vi "Initialize Z Stack.vi"(6 "error in (no error)":errorcluster, 8 "Zstack Settings in":T1, 9 "Automation State in":T3={"Automation State"=enum."Idle", "Handle out"=0, "ZO State"={"ZO Settings"={"Acquisition Settings"={"Save?"=FALSE, "DCIMG Path"=path "", "Filename"="", "Total Frames"=0, "Sender"=enum."UI"}, "Shift Amplitude"=0.0, "Initial Zernike Vector"=[]}, "Zernike Size"=15, "Points per order"=15, "Zernike State"=enum."Idle", "Zernike Vectors"=[], "Total Frames"=15, "Current Frame"=15}, "Zstack State"={"Zstack Settings"={"Acquisition Settings"={"Save?"=FALSE, "DCIMG Path"=path "", "Filename"="", "Total Frames"=0, "Sender"=enum."UI"}, "XYZ start"=[], "XYZ end"=[]}, "Zstack State"=enum."Idle", "Stack Coordinates"=[], "Total Frames"=15, "Current Frame"=15}}) -> (0 "error out":errorcluster, 3 "Automation State Out":T3={"Automation State"=enum."Idle", "Handle out"=0, "ZO State"={"ZO Settings"={"Acquisition Settings"={"Save?"=FALSE, "DCIMG Path"=path "", "Filename"="", "Total Frames"=0, "Sender"=enum."UI"}, "Shift Amplitude"=0.0, "Initial Zernike Vector"=[]}, "Zernike Size"=15, "Points per order"=15, "Zernike State"=enum."Idle", "Zernike Vectors"=[], "Total Frames"=15, "Current Frame"=15}, "Zstack State"={"Zstack Settings"={"Acquisition Settings"={"Save?"=FALSE, "DCIMG Path"=path "", "Filename"="", "Total Frames"=0, "Sender"=enum."UI"}, "XYZ start"=[], "XYZ end"=[]}, "Zstack State"=enum."Idle", "Stack Coordinates"=[], "Total Frames"=15, "Current Frame"=15}})   [LabVIEW 2015, in "Automation.lvlib"]
uses:
  Automation.lvlib
  Automation State.ctl
  Automation Loop State.ctl
  ZO State.ctl
  ZO Settings.ctl
  Camera/Acquisition Settings.ctl
  Zstack State.ctl
  Zstack Settings.ctl
  Camera/Camera.lvlib
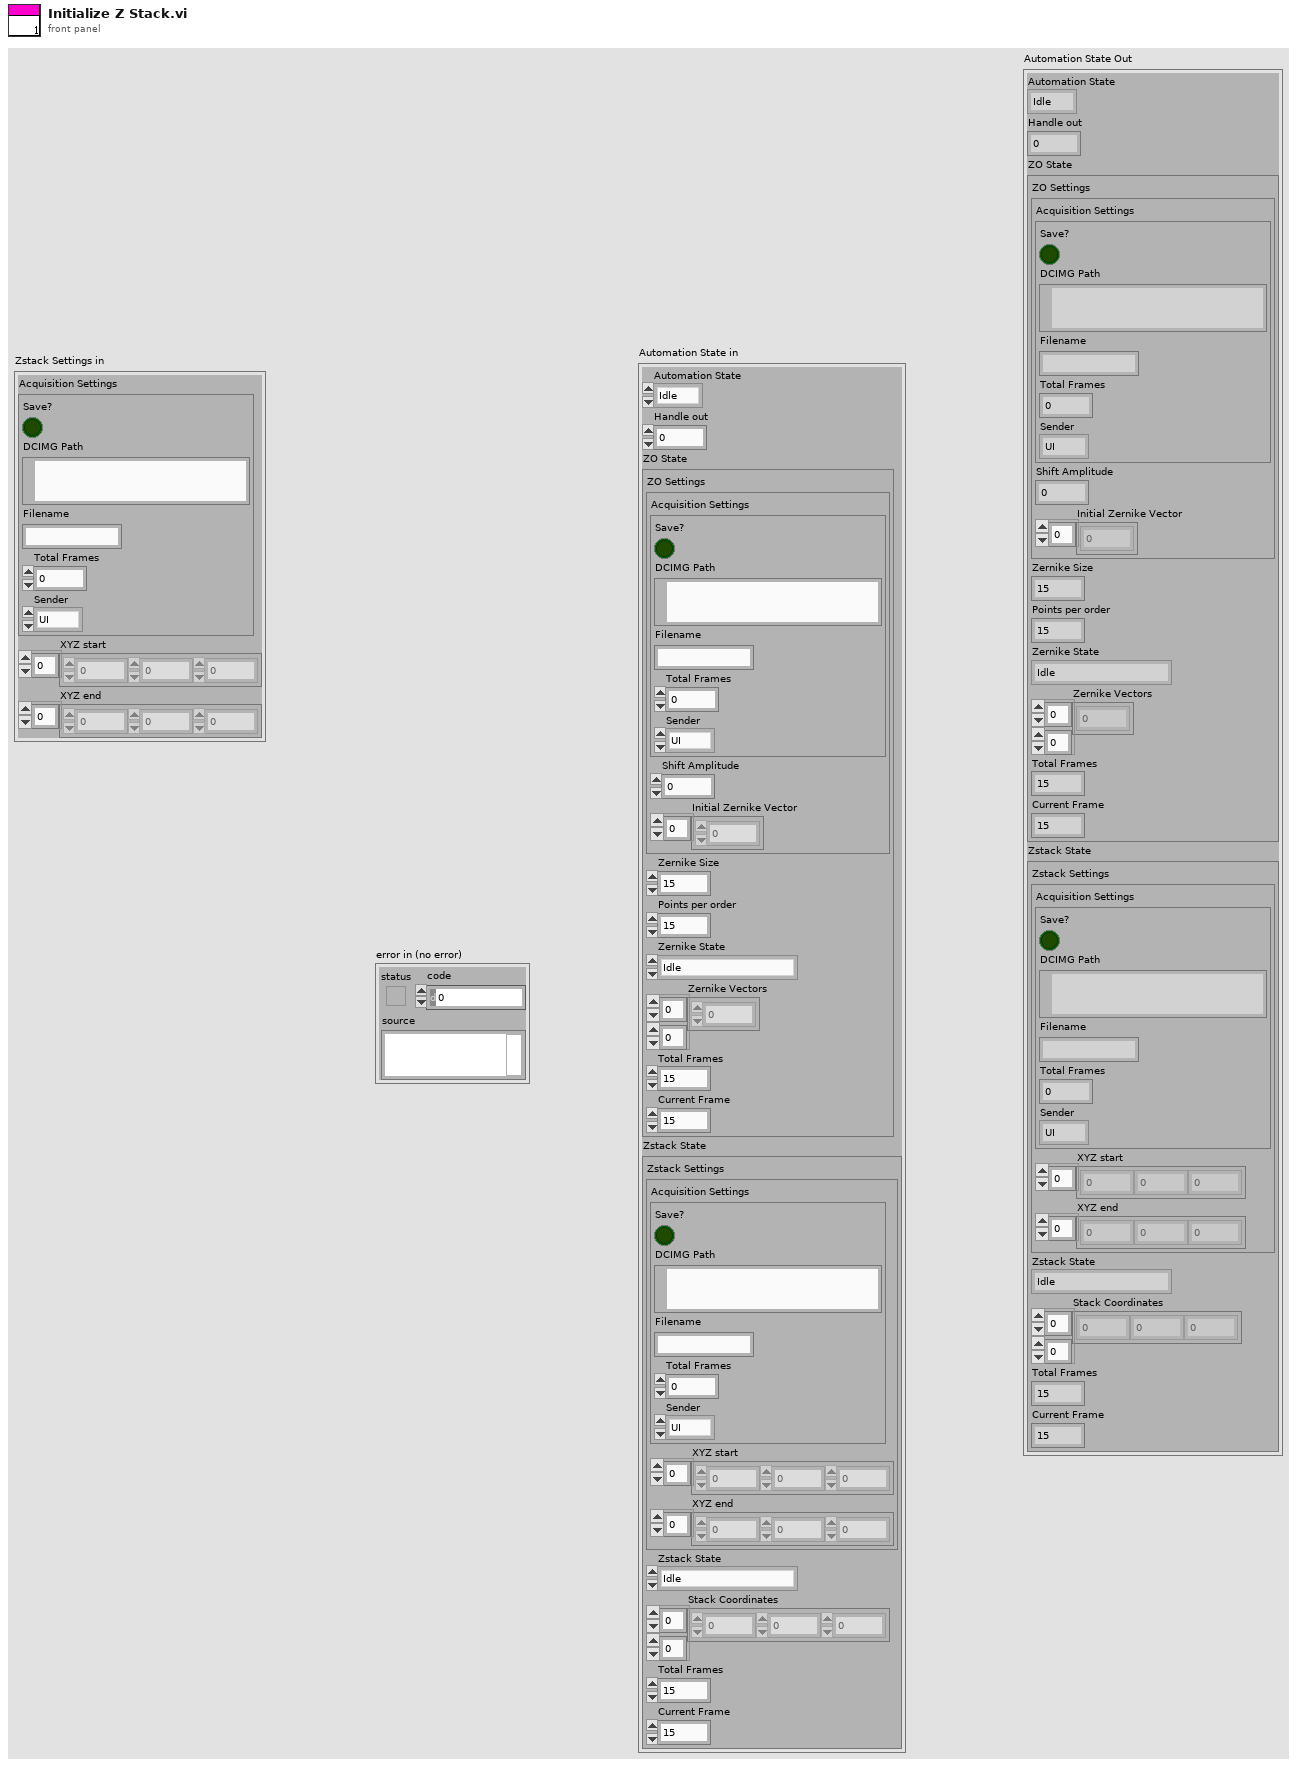
[diagram p1: front panel]
types:
  T1 = typedef "Automation.lvlib/Zstack Settings.ctl" = cluster{"Acquisition Settings":T2, "XYZ start":dbl[], "XYZ end":dbl[]}
  T2 = typedef "Camera.lvlib/Acquisition Settings.ctl" = cluster{"Save?":bool, "DCIMG Path":path, "Filename":string, "Total Frames":i32, "Sender":enum16{"UI", "Automation"}}
  T3 = typedef "Automation.lvlib/Automation State.ctl" = cluster{"Automation State":T4, "Handle out":u32, "ZO State":T5, "Zstack State":T7}
  T4 = typedef "Automation.lvlib/Automation Loop State.ctl" = enum16{"Idle", "Zernike Optimization", "Z Stack"}
  T5 = typedef "Automation.lvlib/ZO State.ctl" = cluster{"ZO Settings":T6, "Zernike Size":i32, "Points per order":i32, "Zernike State":enum16{"Idle", "Waiting for Camera Init.", "Wait for camera frame", "Ready for new mirror config"}, "Zernike Vectors":dbl[][], "Total Frames":i32, "Current Frame":i32}
  T6 = typedef "Automation.lvlib/ZO Settings.ctl" = cluster{"Acquisition Settings":T2, "Shift Amplitude":dbl, "Initial Zernike Vector":dbl[]}
  T7 = typedef "Automation.lvlib/Zstack State.ctl" = cluster{"Zstack Settings":T1, "Zstack State":enum16{"Idle", "Waiting for Camera Init.", "Wait for camera frame", "Ready for new position"}, "Stack Coordinates":dbl[][], "Total Frames":i32, "Current Frame":i32}
  T8 = enum16{"Idle", "Waiting for Camera Init.", "Wait for camera frame", "Ready for new position"}
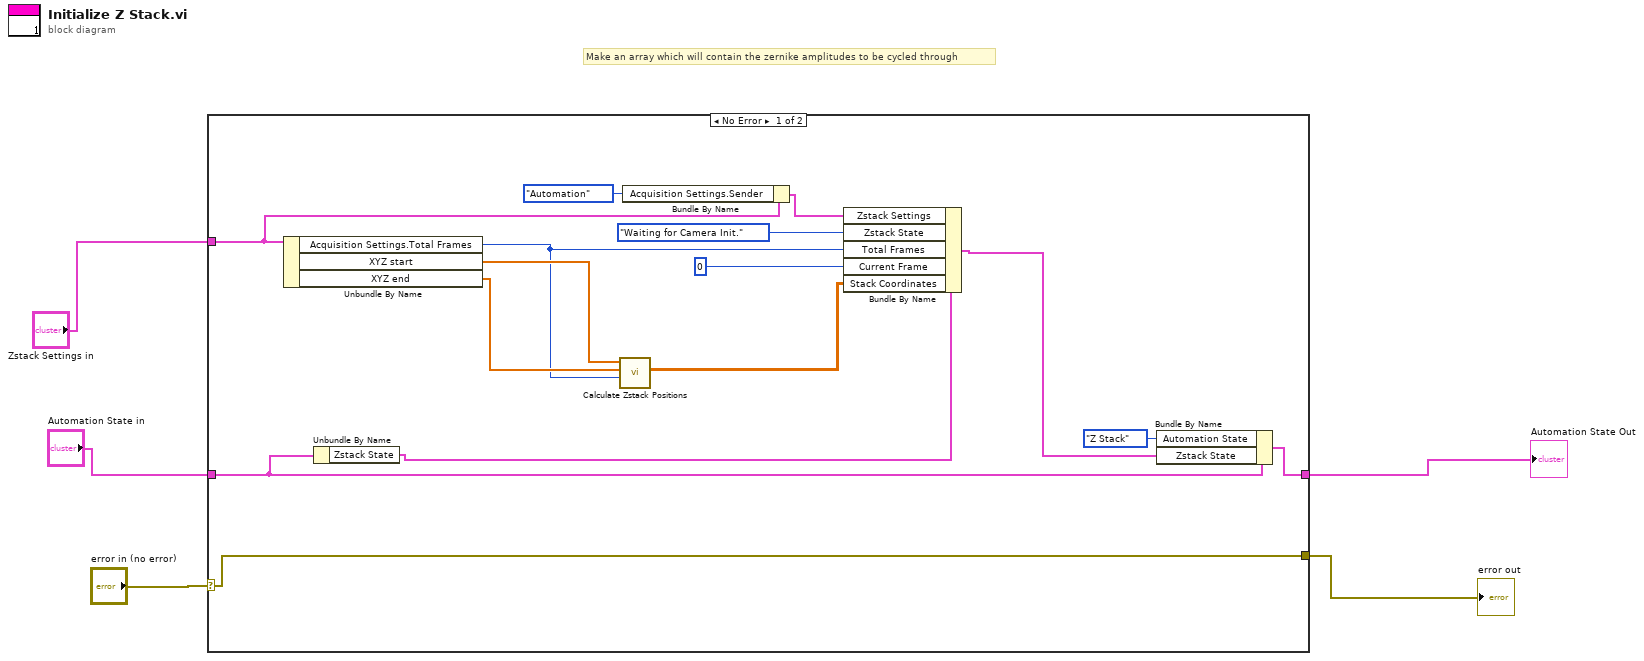
[diagram p0: block diagram]
diagram:
  # "Make an array which will contain the zernike amplitudes to be cycled through"
  n1 = case shown="No Error" "error in (no error)" {
    selector: "error in (no error)" -> [w20 w22]
    tunnel: [w20 w22] -> w4
    tunnel: "Zstack Settings in" -> [w8 _]
    tunnel: [w16 w21] -> w3
    tunnel: "Automation State in" -> [w17 w21]
    frame No Error {
      n2 = Unbundle By Name(w8) -> ("Acquisition Settings.Total Frames"=w11:i32, "XYZ start"=w14:dbl[], "XYZ end"=w13:dbl[])
      n3 = Unbundle By Name(w17) -> ("Zstack State"=w19:T7)
      n4 = call "Calculate Zstack Positions.vi"("Number of Frames"=w11, "XYZ end in"=w13, "XYZ start in"=w14) -> ("Stack Coordinates Out"=w12:dbl[][])  [unwired: 8 in]
      n5 = Bundle By Name(cluster=w8, "Acquisition Settings.Sender"=enum16{"UI", "Automation"}."Automation") -> (w7:T1)
      n6 = Bundle By Name(cluster=w19, "Zstack Settings"=w7, "Zstack State"=T8."Waiting for Camera Init.", "Total Frames"=w11, "Current Frame"=0, "Stack Coordinates"=w12) -> (w15:T7)
      n7 = Bundle By Name(cluster=w17, "Automation State"=Automation_Loop_State."Z Stack", "Zstack State"=w15) -> (w16:T3)
    }
    frame Error {
    }
  }
  "error out" <- w4
  "Automation State Out" <- w3
